vi "omni2 (trig).vi"   [LabVIEW 2012, in "Omni2013.lvrbt"]
uses:
  Omni2013.lvrbt
  <vilib>/NXT/Hardware/Plugins/Tetrix DC Motor/TetrixDCMotorAddress.ctl
  <vilib>/NXT/Hardware/Plugins/Tetrix 180 deg Servo/Tetrix180ServoAddress.ctl
  <vilib>/NXT/Dual Mode Library/Display/drawNumber_float.vi
  <vilib>/NXT/Dual Mode Library/prims/inRangeAndCoerce/inRangeAndCoerce_float.vi
  <vilib>/NXT/NXTIO Xnodes/NXTIONodeSubVIs/TETRIX IO Move DC Motors.vi
  <vilib>/NXT/NXTIO Xnodes/NXTIONodeSubVIs/TETRIX IO Move Servos.vi
  <vilib>/NXT/Dual Mode Library/Display/drawText_Center.vi
  <vilib>/NXT/NXTIO Xnodes/AddressXNode/NXTIOAddress.xnode
  <vilib>/NXT/NXTIO Xnodes/NXTIOXNode/NXTIO.xnode
  <vilib>/NXT/Subs/LVHSConnector.ctl
  <vilib>/NXT/LegoClasses/BrickReference/BrickReference.lvclass
types:
  T1 = typedef "TetrixDCMotorAddress.ctl" = i16
  T2 = cluster{"TetrixDCMotor":T1, "TetrixDCMotor 2":T1}
  T3 = typedef "LVHSConnector.ctl" = refnum<class "BrickReference.lvclass">
  T4 = typedef "FTC ControllerState.ctl" = cluster{"Left X":i8, "Left Y":i8, "Right X":i8, "Right Y":i8, "Button Encoding 9-12":u8, "Button Encoding 1-8":u8, "POV":T5}
  T5 = typedef "FTC POVState.ctl" = i8
  T6 = typedef "FTC ButtonEventType.ctl" = enum16{"Pressed", "Released"}
  T7 = cluster{"Button ID":enum16{"None", "Button 1", "Button 2", "Button 3", "Button 4", "Button 5", "Button 6", "Button 7", "Button 8", "Button 9", "Button 10", "Button 11", "Button 12", "POV Up", "POV Up Right", "POV Right", "POV Down Right", "POV Down", "POV Down Left", "POV Left", "POV Up Left"}, "Event Type":T6}[]
  T8 = enum16{"None", "Button 1", "Button 2", "Button 3", "Button 4", "Button 5", "Button 6", "Button 7", "Button 8", "Button 9", "Button 10", "Button 11", "Button 12", "POV Up", "POV Up Right", "POV Right", "POV Down Right", "POV Down", "POV Down Left", "POV Left", "POV Up Left"}
  T9 = typedef "Tetrix180ServoAddress.ctl" = i16
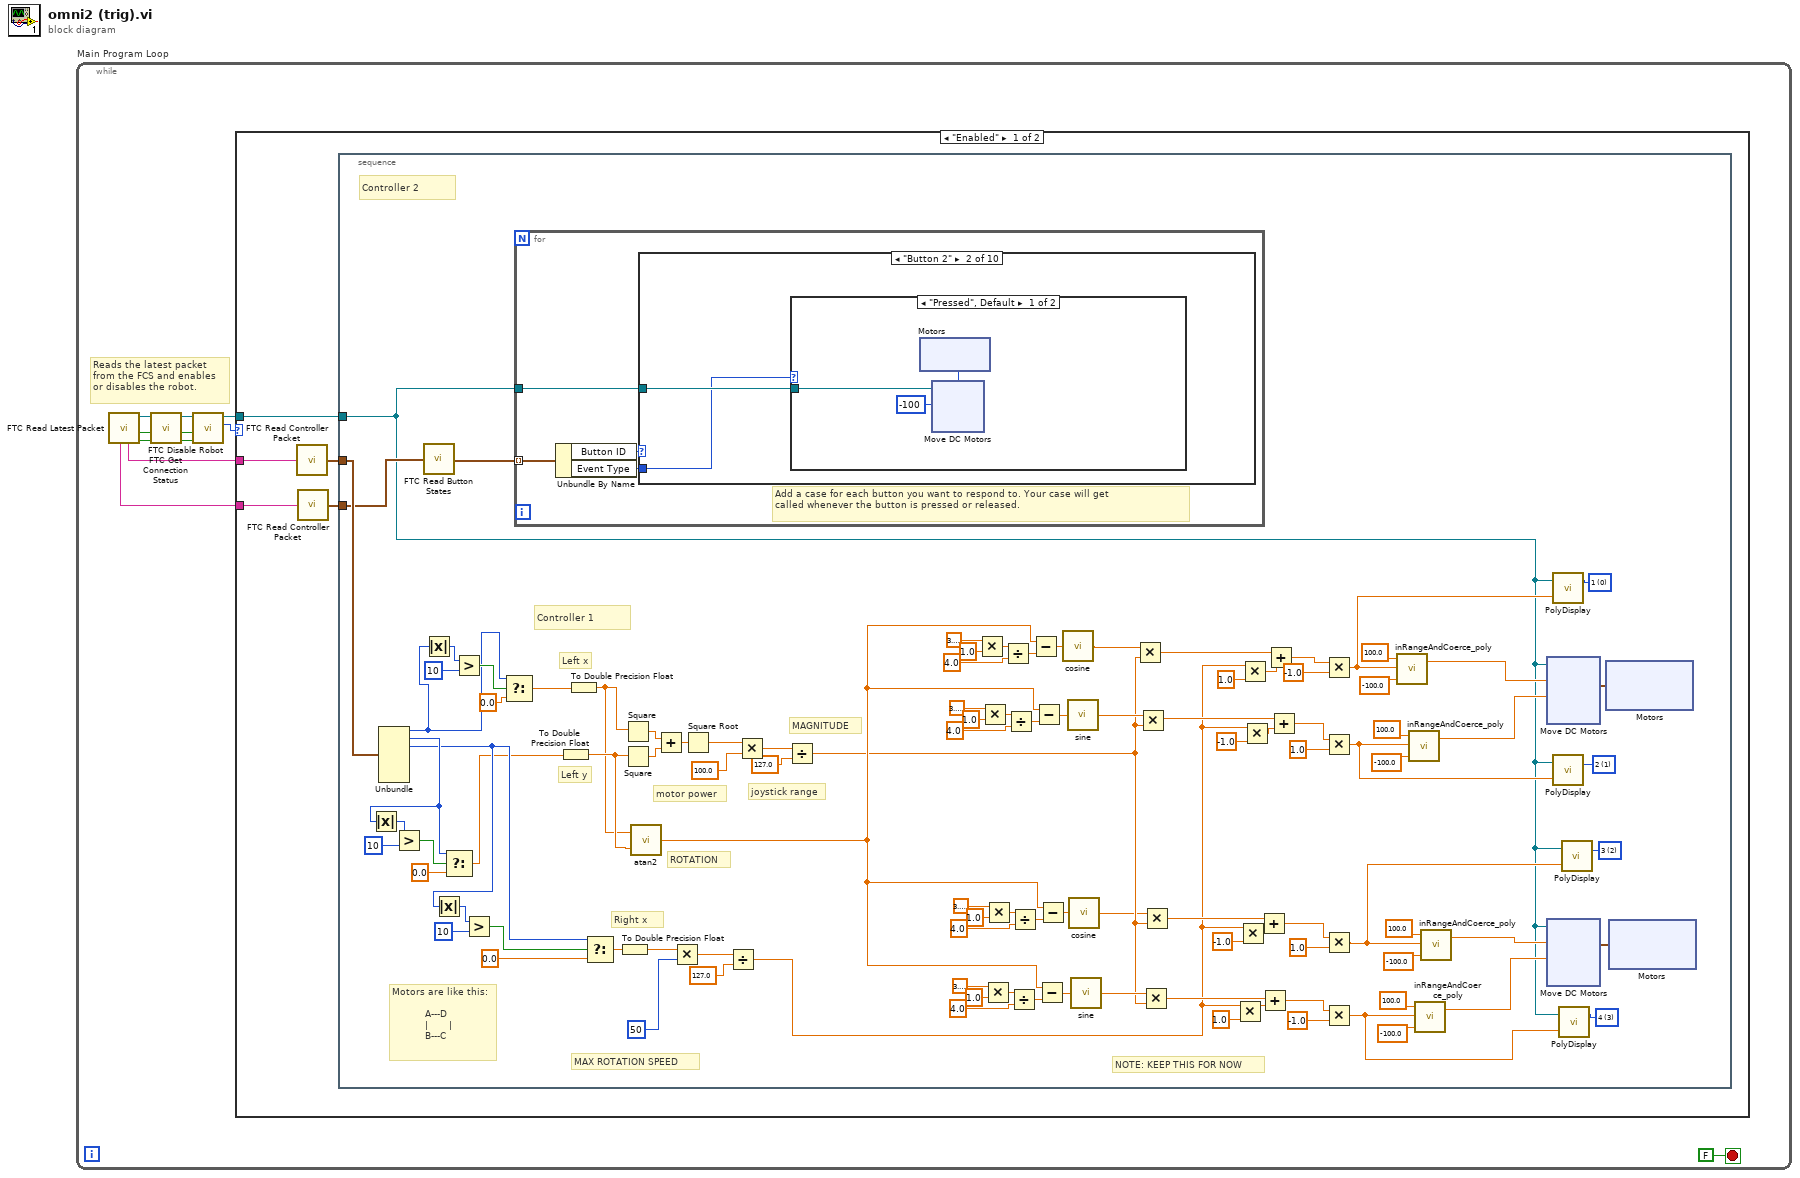
[diagram p0: block diagram]
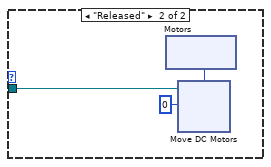
[diagram p3: hidden frame]
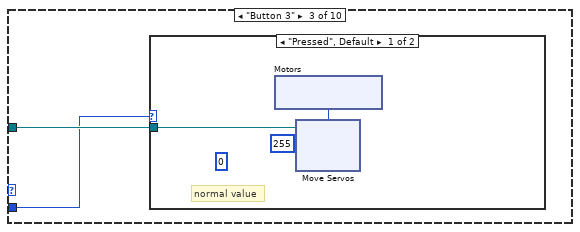
[diagram p4: hidden frame]
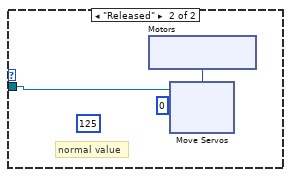
[diagram p5: hidden frame]
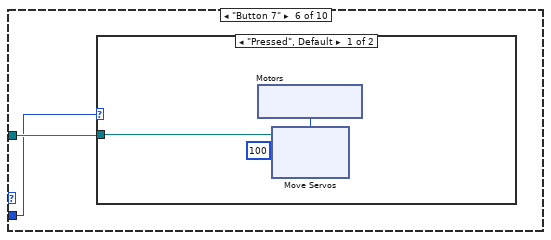
[diagram p8: hidden frame]
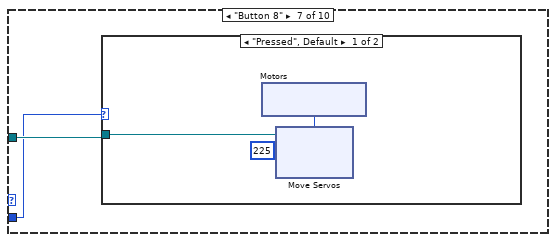
[diagram p10: hidden frame]
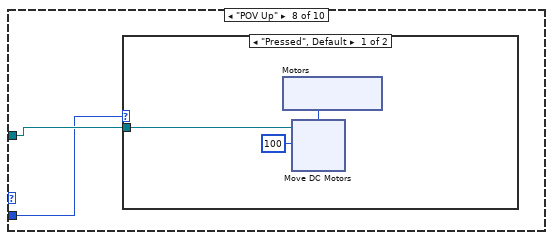
[diagram p12: hidden frame]
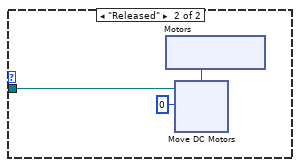
[diagram p13: hidden frame]
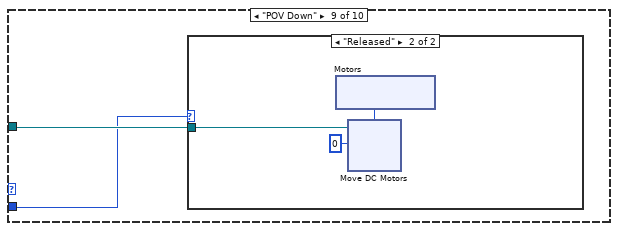
[diagram p14: hidden frame]
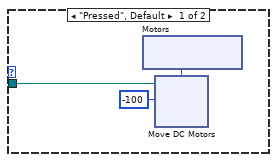
[diagram p15: hidden frame]
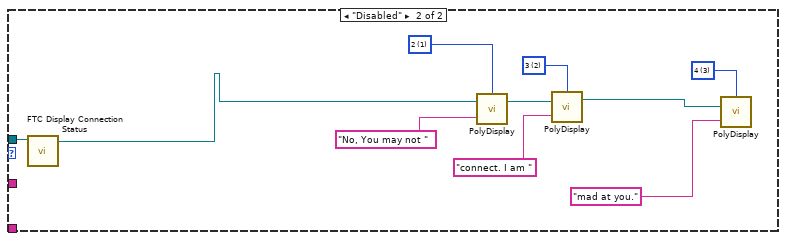
[diagram p17: hidden frame]
diagram:
  n1 = while "Main Program Loop" {
    stop <- FALSE stop-if-true
    # "Reads the latest packet\nfrom the FCS and enables\nor disables the robot."
    n2 = call <vilib>:"FTC Read Latest Packet.vi"() -> ("Packet Received?"=w9:bool, "Stopped?"=w6:bool, "NXT"=w8:T3, "Controller 1"=w10:string, "Controller 2"=w1:string)  [unwired: 6 in, 1 out]
    n3 = call <vilib>:"FTC Get Connection Status.vi"("Packet Received?"=w9, "Stopped?"=w6, "NXT"=w8) -> ("Online?"=w3:bool, "Stopped?"=w4:bool, "NXT"=w5:T3)  [unwired: 5 in]
    n4 = call <vilib>:"FTC Disable Robot.vi"("Online?"=w3, "Stopped?"=w4, "NXT"=w5) -> ("Enabled?"=w7:enum16{"Disabled", "Enabled"}, "NXT"=w2:T3)  [unwired: 3 in]
    n5 = case "disableCase" shown="\"Enabled\"" w7 {
      tunnel: w10 -> [w16 _]
      tunnel: w2 -> [w14 w282]
      tunnel: w1 -> [w13 _]
      frame "Enabled" {
        n6 = call <vilib>:"FTC Read Controller Packet.vi"("Packet"=w16) -> ("Controller State"=w15:T4)  [unwired: 4 in]
        n7 = call <vilib>:"FTC Read Controller Packet.vi"("Packet"=w13) -> ("Controller State"=w12:T4)  [unwired: 4 in]
        n8 = stacked-sequence "controller1Actions" {
          tunnel: w15 -> [w121]
          tunnel: w14 -> [w18]
          tunnel: w12 -> [w101]
          frame #0 {
            w124 = i16 0 items=["1", "2", "3", "4", "5", "6", "7", "8"] ("Line")
            w123 = i16 3 items=["1", "2", "3", "4", "5", "6", "7", "8"] ("Line")
            w118 = i16 2 items=["1", "2", "3", "4", "5", "6", "7", "8"] ("Line")
            w122 = i16 1 items=["1", "2", "3", "4", "5", "6", "7", "8"] ("Line")
            # "NOTE: KEEP THIS FOR NOW"
            # "MAX ROTATION SPEED"
            # "ROTATION"
            # "MAGNITUDE"
            # "joystick range"
            # "motor power"
            # "Controller 1"
            # "Motors are like this:\n\n           A---D\n           |       |\n           B---C"
            # "Left y"
            # "Right x"
            # "Left x"
            # "Controller 2"
            n9 = Unbundle(w121) -> ("Left X"=w107:i8, "Left Y"=w105:i8, "Right X"=w103:i8)  [unwired: 4 out]
            n10 = Absolute Value(x=w105) -> (abs(x)=w106:i8)
            n11 = Greater?(x=w106, y=i8 10) -> (0:w112:bool)
            n12 = call <vilib>:"FTC Read Button States.vi"("Controller State"=w101) -> ("Button Events"=w102:T7)  [unwired: 2 in, 1 out]
            n13 = Absolute Value(x=w107) -> (abs(x)=w108:i8)
            n14 = Absolute Value(x=w103) -> (abs(x)=w104:i8)
            n15 = Select(t=w105, s=w112, f=0.0) -> (s? t:f=w33:dbl)
            n16 = Greater?(x=w108, y=i8 10) -> (0:w115:bool)
            n17 = Greater?(x=w104, y=i8 10) -> (0:w109:bool)
            n18 = Select(t=w107, s=w115, f=0.0) -> (s? t:f=w32:dbl)
            n19 = for "buttonAction" {
              tunnel: w102 -> [w148] mode=indexing
              tunnel: w18 -> [w147]
              # "Add a case for each button you want to respond to. Your case will get \ncalled whenever the button is pressed or released."
              n20 = Unbundle By Name(w148) -> ("Button ID"=w150:T8, "Event Type"=w149:T6)
              n21 = case "EventCase1" shown="\"Button 2\"" w150 {
                tunnel: w149 -> [_ w151 w175 _ _ w199 w212 w225 w249 _]
                tunnel: w147 -> [_ w152 w176 _ _ w200 w213 w226 w250 _]
                frame "Button 1" {
                }
                frame "Button 2" {
                  n22 = case shown="\"Pressed\", Default" w151 {
                    tunnel: w152 -> [w154 w165]
                    frame "Pressed", Default {
                      n23 = xnode "Motors"() -> ("Motor"=w153:T1)
                      n24 = xnode "Move DC Motors"("Power/Speed 1"=i8 -100, "Motors"=w153, "NXT"=w154) -> ()  [unwired: 1 out]
                    }
                    frame "Released" {
                      n25 = xnode "Motors"() -> ("Motor"=w164:T1)
                      n26 = xnode "Move DC Motors"("Power/Speed 1"=i8 0, "Motors"=w164, "NXT"=w165) -> ()  [unwired: 1 out]
                    }
                  }
                }
                frame "Button 3" {
                  n27 = case shown="\"Pressed\", Default" w175 {
                    tunnel: w176 -> [w179 w188]
                    frame "Pressed", Default {
                      (unwired) u8 0 ("Position 1")
                      # "normal value"
                      n28 = xnode "Motors"() -> ("Motor"=w177:T9)
                      n29 = xnode "Move Servos"("Position 1"=u8 255, "Servos"=w177, "NXT"=w179) -> ()  [unwired: 1 out]
                    }
                    frame "Released" {
                      (unwired) u8 125 ("Position 1")
                      # "normal value"
                      n30 = xnode "Motors"() -> ("Motor"=w189:T9)
                      n31 = xnode "Move Servos"("Position 1"=u8 0, "Servos"=w189, "NXT"=w188) -> ()  [unwired: 1 out]
                    }
                  }
                }
                frame "Button 4" {
                }
                frame "Button 5" {
                }
                frame "Button 7" {
                  n32 = case shown="\"Pressed\", Default" w199 {
                    tunnel: w200 -> [w202 _]
                    frame "Pressed", Default {
                      n33 = xnode "Motors"() -> ("Motor"=w203:T9)
                      n34 = xnode "Move Servos"("Position 1"=u8 100, "Servos"=w203, "NXT"=w202) -> ()  [unwired: 1 out]
                    }
                    frame "Released" {
                    }
                  }
                }
                frame "Button 8" {
                  n35 = case shown="\"Pressed\", Default" w212 {
                    tunnel: w213 -> [w214 _]
                    frame "Pressed", Default {
                      n36 = xnode "Motors"() -> ("Motor"=w216:T9)
                      n37 = xnode "Move Servos"("Position 1"=u8 225, "Servos"=w216, "NXT"=w214) -> ()  [unwired: 1 out]
                    }
                    frame "Released" {
                    }
                  }
                }
                frame "POV Up" {
                  n38 = case shown="\"Pressed\", Default" w225 {
                    tunnel: w226 -> [w228 w239]
                    frame "Pressed", Default {
                      n39 = xnode "Motors"() -> ("Motor"=w227:T1)
                      n40 = xnode "Move DC Motors"("Power/Speed 1"=i8 100, "Motors"=w227, "NXT"=w228) -> ()  [unwired: 1 out]
                    }
                    frame "Released" {
                      n41 = xnode "Motors"() -> ("Motor"=w238:T1)
                      n42 = xnode "Move DC Motors"("Power/Speed 1"=i8 0, "Motors"=w238, "NXT"=w239) -> ()  [unwired: 1 out]
                    }
                  }
                }
                frame "POV Down" {
                  n43 = case shown="\"Released\"" w249 {
                    tunnel: w250 -> [w252 w263]
                    frame "Pressed", Default {
                      n44 = xnode "Motors"() -> ("Motor"=w251:T1)
                      n45 = xnode "Move DC Motors"("Power/Speed 1"=i8 -100, "Motors"=w251, "NXT"=w252) -> ()  [unwired: 1 out]
                    }
                    frame "Released" {
                      n46 = xnode "Motors"() -> ("Motor"=w262:T1)
                      n47 = xnode "Move DC Motors"("Power/Speed 1"=i8 0, "Motors"=w262, "NXT"=w263) -> ()  [unwired: 1 out]
                    }
                  }
                }
                frame Default {
                  # "No Action"
                }
              }
            }
            n48 = To Double Precision Float(number=w33) -> (double precision float=w35:dbl)
            n49 = To Double Precision Float(number=w32) -> (double precision float=w34:dbl)
            n50 = Select(t=w103, s=w109, f=0.0) -> (s? t:f=w53:dbl)
            n51 = To Double Precision Float(number=w53) -> (double precision float=w52:dbl)
            n52 = Square(x=w34) -> (x^2=w99:dbl)
            n53 = Square(x=w35) -> (x^2=w98:dbl)
            n54 = call <vilib>:"atan2.vi"("x"=w35, "y"=w34) -> ("atan2(y,x)"=w63:sgl)
            n55 = Add(x=w99, y=w98) -> (x+y=w100:dbl)
            n56 = Multiply(x=w52, y=50) -> (x*y=w31:dbl)
            n57 = Square Root(x=w100) -> (sqrt(x)=w95:dbl)
            n58 = Divide(x=w31, y=127.0) -> (x/y=w17:dbl)
            n59 = Multiply(x=w95, y=100.0) -> (x*y=w94:dbl)
            n60 = Divide(x=w94, y=127.0) -> (x/y=w54:dbl)
            n61 = Multiply(x=3.141592653589793, y=1.0) -> (x*y=w89:dbl)
            n62 = Multiply(x=3.141592653589793, y=1.0) -> (x*y=w83:dbl)
            n63 = Multiply(x=3.141592653589793, y=1.0) -> (x*y=w65:dbl)
            n64 = Multiply(x=3.141592653589793, y=1.0) -> (x*y=w77:dbl)
            n65 = Divide(x=w89, y=4.0) -> (x/y=w92:dbl)
            n66 = Divide(x=w83, y=4.0) -> (x/y=w87:dbl)
            n67 = Divide(x=w65, y=4.0) -> (x/y=w69:dbl)
            n68 = Divide(x=w77, y=4.0) -> (x/y=w80:dbl)
            n69 = Subtract(x=w63, y=w92) -> (x-y=w39:dbl)
            n70 = Subtract(x=w63, y=w87) -> (x-y=w86:dbl)
            n71 = Subtract(x=w63, y=w69) -> (x-y=w68:dbl)
            n72 = Subtract(x=w63, y=w80) -> (x-y=w37:dbl)
            n73 = call <vilib>:"cosine.vi"("x"=w39) -> ("cos(x)"=w38:sgl)
            n74 = call <vilib>:"sine.vi"("x"=w86) -> ("sin(x)"=w82:sgl)
            n75 = call <vilib>:"cosine.vi"("x"=w37) -> ("cos(x)"=w36:sgl)
            n76 = call <vilib>:"sine.vi"("x"=w68) -> ("sin(x)"=w64:sgl)
            n77 = Multiply(x=w38, y=w54) -> (x*y=w62:dbl)
            n78 = Multiply(x=w82, y=w54) -> (x*y=w59:dbl)
            n79 = Multiply(x=w64, y=w54) -> (x*y=w61:dbl)
            n80 = Multiply(x=w36, y=w54) -> (x*y=w60:dbl)
            n81 = Multiply(x=w17, y=1.0) -> (x*y=w29:dbl)
            n82 = Multiply(x=w17, y=-1.0) -> (x*y=w27:dbl)
            n83 = Multiply(x=w17, y=1.0) -> (x*y=w23:dbl)
            n84 = Multiply(x=w17, y=-1.0) -> (x*y=w25:dbl)
            n85 = Add(x=w60, y=w27) -> (x+y=w57:dbl)
            n86 = Add(x=w61, y=w29) -> (x+y=w58:dbl)
            n87 = Add(x=w62, y=w23) -> (x+y=w55:dbl)
            n88 = Add(x=w59, y=w25) -> (x+y=w56:dbl)
            n89 = Multiply(x=w55, y=-1.0) -> (x*y=w20:dbl)
            n90 = Multiply(x=w56, y=1.0) -> (x*y=w19:dbl)
            n91 = Multiply(x=w57, y=1.0) -> (x*y=w21:dbl)
            n92 = Multiply(x=w58, y=-1.0) -> (x*y=w22:dbl)
            n93 = call-poly <vilib>:"inRangeAndCoerce_poly.vi"("lower limit"=-100.0, "x"=w20, "upper limit"=100.0) -> ("coerced(x)"=w49:dbl)  [unwired: 1 out]
            n94 = call-poly <vilib>:"inRangeAndCoerce_poly.vi"("lower limit"=-100.0, "x"=w19, "upper limit"=100.0) -> ("coerced(x)"=w46:dbl)  [unwired: 1 out]
            n95 = call-poly <vilib>:"inRangeAndCoerce_poly.vi"("lower limit"=-100.0, "x"=w22, "upper limit"=100.0) -> ("coerced(x)"=w41:dbl)  [unwired: 1 out]
            n96 = call-poly <vilib>:"inRangeAndCoerce_poly.vi"("lower limit"=-100.0, "x"=w21, "upper limit"=100.0) -> ("coerced(x)"=w40:dbl)  [unwired: 1 out]
            n97 = call-poly <vilib>:"PolyDisplay.vi"("number"=w20, "NXT"=w18, "Line"=w124) -> ()  [unwired: 1 in, 1 out]
            n98 = call-poly <vilib>:"PolyDisplay.vi"("number"=w19, "NXT"=w18, "Line"=w122) -> ()  [unwired: 1 in, 1 out]
            n99 = call-poly <vilib>:"PolyDisplay.vi"("number"=w22, "NXT"=w18, "Line"=w123) -> ()  [unwired: 1 in, 1 out]
            n100 = call-poly <vilib>:"PolyDisplay.vi"("number"=w21, "NXT"=w18, "Line"=w118) -> ()  [unwired: 1 in, 1 out]
            n101 = xnode "Motors"() -> ("Motor"=w120:cluster{"TetrixDCMotor":T1, "TetrixDCMotor":T1})
            n102 = xnode "Move DC Motors"("Power/Speed 2"=w46, "Power/Speed 1"=w49, "Motors"=w120, "NXT"=w18) -> ()  [unwired: 1 out]
            n103 = xnode "Motors"() -> ("Motor"=w119:cluster{"TetrixDCMotor":T1, "TetrixDCMotor":T1})
            n104 = xnode "Move DC Motors"("Power/Speed 2"=w41, "Power/Speed 1"=w40, "Motors"=w119, "NXT"=w18) -> ()  [unwired: 1 out]
          }
        }
      }
      frame "Disabled" {
        w275 = i16 3 items=["1", "2", "3", "4", "5", "6", "7", "8"] ("Line")
        w281 = i16 2 items=["1", "2", "3", "4", "5", "6", "7", "8"] ("Line")
        w277 = i16 1 items=["1", "2", "3", "4", "5", "6", "7", "8"] ("Line")
        n105 = call <vilib>:"FTC Display Connection Status.vi"("NXT"=w282) -> ("NXT"=w276:T3)  [unwired: 10 in]
        n106 = call-poly <vilib>:"PolyDisplay.vi"("Text"="No, You may not ", "NXT"=w276, "Line"=w277) -> ("NXT"=w279:T3)  [unwired: 1 in]
        n107 = call-poly <vilib>:"PolyDisplay.vi"("Text"="connect. I am ", "NXT"=w279, "Line"=w281) -> ("NXT"=w274:T3)  [unwired: 1 in]
        n108 = call-poly <vilib>:"PolyDisplay.vi"("Text"="mad at you.", "NXT"=w274, "Line"=w275) -> ()  [unwired: 1 in, 1 out]
      }
    }
  }
